vi "set_settings_cluster.vi"(8 "error in (no error)":errorcluster, 10 "settings cluster variant":variant, 11 "ImagingModeDL090130Frame in":refnum<class "ImagingModeDL090130Frame.lvclass">) -> (0 "error out":errorcluster, 3 "ImagingModeDL090130Frame out":refnum<class "ImagingModeDL090130Frame.lvclass">)   [LabVIEW 2010, in "ImagingModeDL090130Frame.lvclass"]
uses:
  ImagingModeDL090130Frame.lvclass
  ImagingModeDL090130Frame.lvclass/ImagingModeDL090130Frame.ctl
  common/xcontrols/XIntensityCompensation/XIntensityCompensation/XIntensityCompensation.xctl
  common/classes/ErrorController/ErrorController/class_data.vi
  common/classes/ErrorController/ErrorController/ErrorController.lvclass
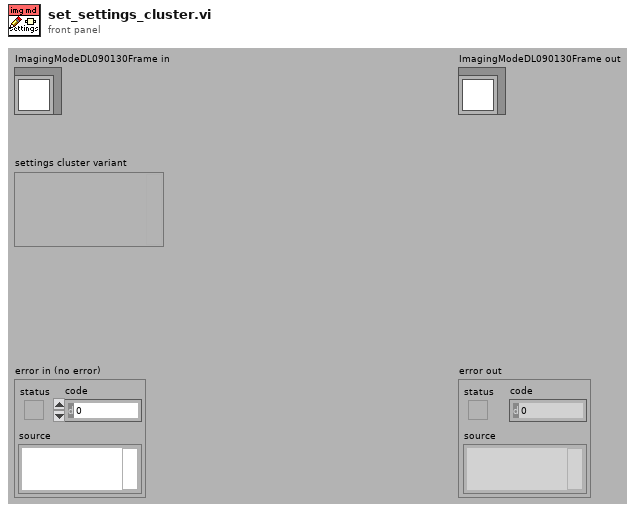
[diagram p1: front panel]
types:
  T1 = typedef "ImagingModeDL090130Frame.lvclass/settings_cluster.ctl" = cluster{"FrameSettings":cluster{"ResolutionX":i32, "ResolutionY":i32, "AspectRatioX":dbl, "AspectRatioY":dbl, "FrameScanRate":dbl[unit]}, "StackSettings":cluster{"Frames":i32, "AveragingRepetitions":i32, "StepSize":dbl[unit], "ReturnToOrigin":bool, "translation mode":T2, "depth/intensity points":cluster{"depth":dbl[unit], "intensity":dbl}[]}}
  T2 = typedef "ImagingModeDL090130Frame.lvclass/translation_mode_enum.ctl" = enum16{"scanHead", "stage"}
  T3 = typedef "ImagingModeDL090130Frame.lvclass/control_refs.ctl" = cluster{"resolution controls":cluster{"x pixels":refnum<vi>, "y pixels":refnum<vi>, "ratio x factor":refnum<vi>, "ratio y factor":refnum<vi>}, "speed controls":cluster{"pixel dwell time":refnum<vi>, "line scan time":refnum<vi>, "frame rate":refnum<vi>}, "number of frames controls":cluster{"# of frames":refnum<vi>, "duration":refnum<vi>, "# of repetitions":refnum<vi>}, "current value indicators":cluster{"frame #":refnum<vi>, "repetition #":refnum<vi>, "offset":refnum<vi>}, "step controls":cluster{"step size":refnum<vi>, "return to origin?":refnum<vi>, "translation mode":refnum<vi>, "XIntensityCompensation":refnum<vi>}, "settings":refnum<vi>, "defineButton":refnum<vi>, "settings enforced?":refnum<vi>}
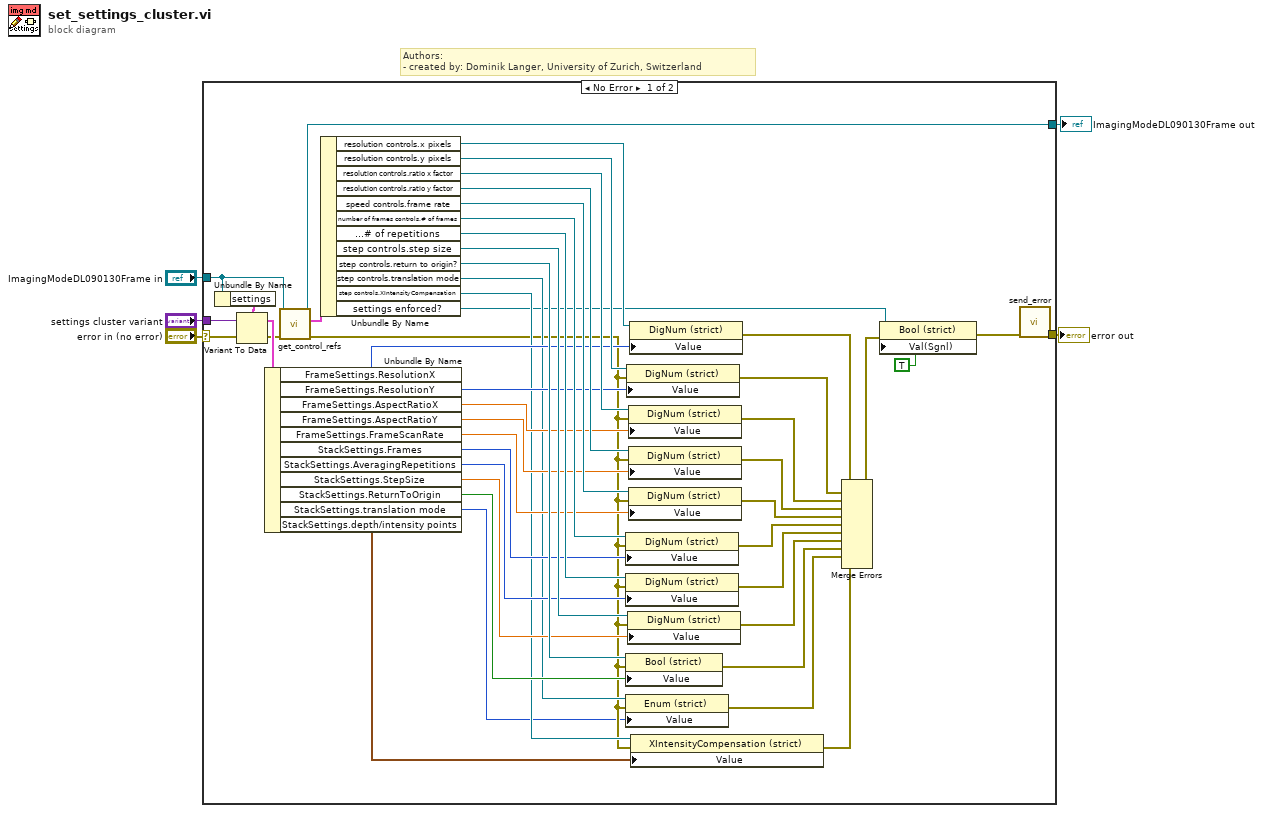
[diagram p0: block diagram]
diagram:
  # "Authors: \n- created by: Dominik Langer, University of Zurich, Switzerland"
  n1 = case shown="No Error" "error in (no error)" {
    selector: "error in (no error)" -> [w29 w54]
    tunnel: [w33 w54] -> w4
    tunnel: [w31 w53] -> w3
    tunnel: "ImagingModeDL090130Frame in" -> [w27 w53]
    tunnel: "settings cluster variant" -> [w28 _]
    frame No Error {
      n2 = Unbundle By Name(w27) -> ("settings"=w26:T1)
      n3 = Variant To Data(error in=w29, Variant=w28, type=w26) -> (error out=w32:errorcluster, data=w43:T1)
      n4 = Unbundle By Name(w43) -> ("FrameSettings.ResolutionX"=w42:i32, "FrameSettings.ResolutionY"=w41:i32, "FrameSettings.AspectRatioX"=w40:dbl, "FrameSettings.AspectRatioY"=w39:dbl, "FrameSettings.FrameScanRate"=w38:dbl[unit], "StackSettings.Frames"=w37:i32, "StackSettings.AveragingRepetitions"=w36:i32, "StackSettings.StepSize"=w35:dbl[unit], "StackSettings.ReturnToOrigin"=w34:bool, "StackSettings.translation mode"=w11:T2, "StackSettings.depth/intensity points"=w12:cluster{"depth":dbl[unit], "intensity":dbl}[])
      n5 = call-dynamic "get_control_refs.vi"("error in (no error)"=w32, "ImagingModeDL090130Frame in"=w27) -> ("error out"=w15:errorcluster, "control refs"=w30:T3, "ImagingModeDL090130Frame out"=w31:refnum<class "ImagingModeDL090130Frame.lvclass">)  [unwired: 7 in]
      n6 = Unbundle By Name(w30) -> ("resolution controls.x pixels"=w52:refnum<vi>, "resolution controls.y pixels"=w51:refnum<vi>, "resolution controls.ratio x factor"=w50:refnum<vi>, "resolution controls.ratio y factor"=w49:refnum<vi>, "speed controls.frame rate"=w48:refnum<vi>, "number of frames controls.# of frames"=w47:refnum<vi>, "number of frames controls.# of repetitions"=w46:refnum<vi>, "step controls.step size"=w45:refnum<vi>, "step controls.return to origin?"=w44:refnum<vi>, "step controls.translation mode"=w17:refnum<vi>, "step controls.XIntensityCompensation"=w16:refnum<vi>, "settings enforced?"=w7:refnum<vi>)
      n7 = property class="DigNum (strict)"(reference=w47, error in=w15, "Value"=w37) -> (error out=w21:errorcluster)  [unwired: 1 out]
      n8 = property class="DigNum (strict)"(reference=w46, error in=w15, "Value"=w36) -> (error out=w20:errorcluster)  [unwired: 1 out]
      n9 = property class="Bool (strict)"(reference=w44, error in=w15, "Value"=w34) -> (error out=w18:errorcluster)  [unwired: 1 out]
      n10 = property class="Enum (strict)"(reference=w17, error in=w15, "Value"=w11) -> (error out=w14:errorcluster)  [unwired: 1 out]
      n11 = property class="DigNum (strict)"(reference=w51, error in=w15, "Value"=w41) -> (error out=w25:errorcluster)  [unwired: 1 out]
      n12 = property class="DigNum (strict)"(reference=w45, error in=w15, "Value"=w35) -> (error out=w19:errorcluster)  [unwired: 1 out]
      n13 = property class="DigNum (strict)"(reference=w50, error in=w15, "Value"=w40) -> (error out=w24:errorcluster)  [unwired: 1 out]
      n14 = property class="DigNum (strict)"(reference=w49, error in=w15, "Value"=w39) -> (error out=w23:errorcluster)  [unwired: 1 out]
      n15 = property class="DigNum (strict)"(reference=w48, error in=w15, "Value"=w38) -> (error out=w22:errorcluster)  [unwired: 1 out]
      n16 = property class="DigNum (strict)"(reference=w52, "Value"=w42) -> (error out=w10:errorcluster)  [unwired: 1 in, 1 out]
      n17 = property class="XIntensityCompensation (strict)"(reference=w16, error in=w15, "Value"=w12) -> (error out=w13:errorcluster)  [unwired: 1 out]
      n18 = Merge Errors(w10, w25, w24, w23, w22, w21, w20, w19, w18, w14, w13) -> (w9:errorcluster)
      n19 = property class="Bool (strict)"(reference=w7, error in=w9, "Val(Sgnl)"=TRUE ("Value (Signaling)")) -> (error out=w8:errorcluster)  [unwired: 1 out]
      n20 = call "send_error.vi"("error in (no error)"=w8) -> ("error out"=w33:errorcluster)  [unwired: 10 in]
    }
    frame Error {
    }
  }
  "error out" <- w4
  "ImagingModeDL090130Frame out" <- w3
